vi "ADD16.vi"(2 "B":bool[](array[boolean])=[FALSE, FALSE, FALSE, FALSE, FALSE, FALSE, FALSE, FALSE, FALSE, FALSE, FALSE, FALSE, FALSE, FALSE, FALSE, FALSE], 3 "A":bool[](array[boolean])=[FALSE, FALSE, FALSE, FALSE, FALSE, FALSE, FALSE, FALSE, FALSE, FALSE, FALSE, FALSE, FALSE, FALSE, FALSE, FALSE], 4 "c in":bool) -> (0 "c out":bool, 1 "S":bool[](array[boolean]))   [LabVIEW 2012]
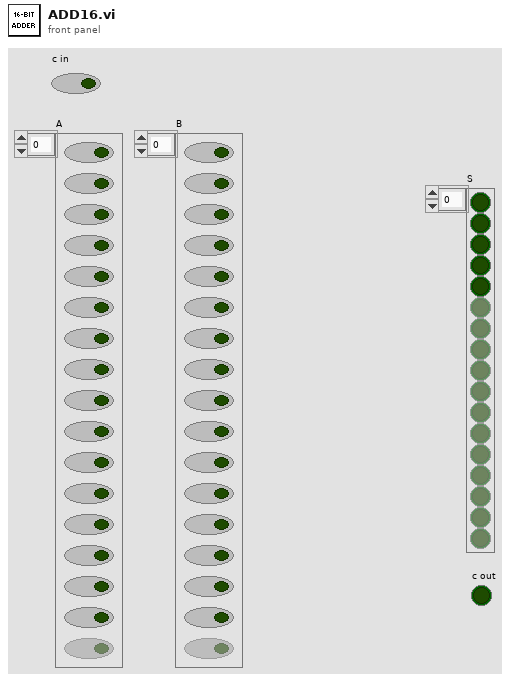
[diagram p1: front panel]
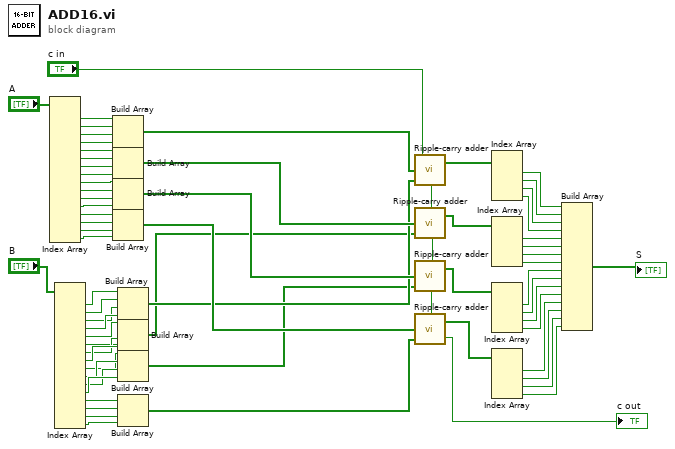
[diagram p0: block diagram]
diagram:
  n1 = Index Array(array="A") -> (element #1=w64:bool, element #2=w63:bool, element #3=w62:bool, element #4=w61:bool, element #5=w60:bool, element #6=w59:bool, element #7=w58:bool, element #8=w57:bool, element #9=w56:bool, element #10=w55:bool, element #11=w54:bool, element #12=w53:bool, element #13=w52:bool, element #14=w51:bool, element #15=w50:bool, element #16=w49:bool)  [unwired: 16 in]
  n2 = Index Array(array="B") -> (element #1=w33:bool, element #2=w34:bool, element #3=w35:bool, element #4=w36:bool, element #5=w37:bool, element #6=w38:bool, element #7=w39:bool, element #8=w40:bool, element #9=w41:bool, element #10=w42:bool, element #11=w43:bool, element #12=w44:bool, element #13=w45:bool, element #14=w46:bool, element #15=w47:bool, element #16=w48:bool)  [unwired: 16 in]
  n3 = Build Array(w64, w63, w62, w61) -> (w31:bool[])
  n4 = Build Array(w60, w59, w58, w57) -> (w30:bool[])
  n5 = Build Array(w56, w55, w54, w53) -> (w29:bool[])
  n6 = Build Array(w52, w51, w50, w49) -> (w28:bool[])
  n7 = Build Array(w33, w34, w35, w36) -> (w27:bool[])
  n8 = Build Array(w37, w38, w39, w40) -> (w26:bool[])
  n9 = Build Array(w41, w42, w43, w44) -> (w25:bool[])
  n10 = Build Array(w45, w46, w47, w48) -> (w24:bool[])
  n11 = call "Ripple-carry adder.vi"("B"=w27, "A"=w31, "c in"="c in") -> ("c out"=w67:bool, "S"=w21:bool[])
  n12 = call "Ripple-carry adder.vi"("B"=w26, "A"=w30, "c in"=w67) -> ("c out"=w66:bool, "S"=w18:bool[])
  n13 = call "Ripple-carry adder.vi"("B"=w25, "A"=w29, "c in"=w66) -> ("c out"=w65:bool, "S"=w19:bool[])
  n14 = call "Ripple-carry adder.vi"("B"=w24, "A"=w28, "c in"=w65) -> ("c out"=→"c out":bool, "S"=w20:bool[])
  n15 = Index Array(array=w21) -> (element #1=w17:bool, element #2=w16:bool, element #3=w15:bool, element #4=w14:bool)  [unwired: 4 in]
  n16 = Index Array(array=w18) -> (element #1=w13:bool, element #2=w12:bool, element #3=w11:bool, element #4=w10:bool)  [unwired: 4 in]
  n17 = Index Array(array=w19) -> (element #1=w9:bool, element #2=w8:bool, element #3=w7:bool, element #4=w6:bool)  [unwired: 4 in]
  n18 = Index Array(array=w20) -> (element #1=w5:bool, element #2=w4:bool, element #3=w3:bool, element #4=w2:bool)  [unwired: 4 in]
  n19 = Build Array(w17, w16, w15, w14, w13, w12, w11, w10, w9, w8, w7, w6, w5, w4, w3, w2) -> (→"S":bool[])
